vi "Self-Test.vi"(8 "error in (no error)":errorcluster, 11 "VISA resource name":refnum<visa-resource-name>) -> (0 "error out":errorcluster, 1 "Self-Test Result Message":string, 2 "Self-Test Result Code":i32, 3 "VISA resource name out":refnum<visa-resource-name>)   [LabVIEW 2023, in "Thermotron 8800.lvlib"]
doc: "Runs the instrument's self-test routine and returns the test results."
uses:
  Thermotron 8800.lvlib
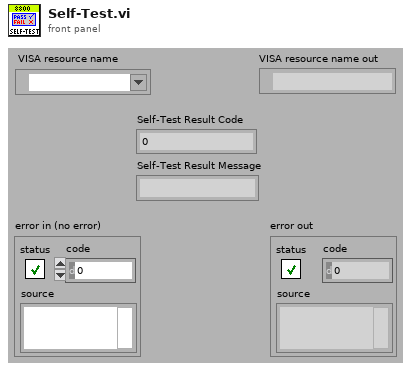
[diagram p1: front panel]
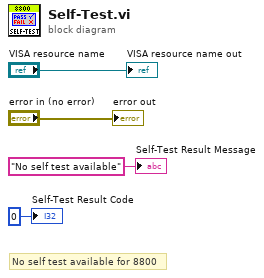
[diagram p0: block diagram]
diagram:
  # "No self test available for 8800"
  "Self-Test Result Message" <- "No self test available" ("Self-Test Result Message")
  "Self-Test Result Code" <- 0 ("Self-Test Result Code")
  "VISA resource name out" <- "VISA resource name"
  "error out" <- "error in (no error)"
